vi "Main.vi"(11 "Module Admin":refnum<class "Delacor_lib_QMH_Cloneable Module Admin.lvclass">) -> ()   [LabVIEW 2020, in "Client HTTP Get.lvlib"]
doc: "This template is based off of the Queued Message Handler design pattern and the Queued Message Handler project template that ships with LabVIEW.\n\nThe main difference is that the queue is private to this module and communication between modules is performed via Broadcast and Request events.\n\nRequest events are wrapped in public API methods and are handled in the Event Handling Loop (EHL) of this VI. Any module can register for Broadcast events sent by this module. The EHL generates messages based on user interface actions.\n\nThe Message Handling Loop (MHL) processes messages generated by the EHL, or by other messages. The messages are string values, so new messages can be added easily to the Message Cases case structure in the MHL. Each message cluster can also provide an optional value for Message Data, which is a variant that can be converted to whatever message-specific data is required.\n_____\nBased on DQMH Project Template 6.0.0.91."
uses:
  Client HTTP Get.lvlib
  <vilib>/Delacor/Delacor QMH/Libraries/Cloneable Module Admin_class/Delacor_lib_QMH_Cloneable Module Admin.lvclass
  C:/Program Files (x86)/National Instruments/LabVIEW 2020/vi.lib/Delacor/Delacor QMH/Libraries/Module Admin_class/Delacor_lib_QMH_Module Admin.lvclass
  Module Data--cluster.ctl
  Do Something Argument--cluster.ctl
  <vilib>/Delacor/Delacor QMH/Libraries/Message Queue_class/Delacor_lib_QMH_Message Queue.lvclass/Delacor_lib_QMH_Message Queue.ctl
  Do Something Else Argument--cluster.ctl
  Do Something Else and Wait for Reply Argument--cluster.ctl
  Do Something Else and Wait (Reply Payload)--cluster.ctl
  <vilib>/Delacor/Delacor QMH/Libraries/Cloneable Module Admin_class/Delacor_lib_QMH_Cloneable Module Admin.lvclass/Delacor_lib_QMH_Cloneable Module Admin.ctl
  Stop Argument--cluster.ctl
  <vilib>/Delacor/Delacor QMH/Libraries/Module Admin_class/Delacor_lib_QMH_Module Admin.lvclass/Delacor_lib_QMH_Module Admin.ctl
  <vilib>/Delacor/Delacor QMH/Libraries/Message Queue_class/Delacor_lib_QMH_Enqueue Message (Single).vi
  <vilib>/Delacor/Delacor QMH/Libraries/Cloneable Module Admin_class/Delacor_lib_QMH_Get Module ID.vi
  <vilib>/Delacor/Delacor QMH/Libraries/Module Admin_class/Delacor_lib_QMH_Get External Launch.vi
  <vilib>/Utility/error.llb/Error Cluster From Error Code.vi
  <vilib>/ErrorRing/Error Ring.xnode
  <vilib>/Delacor/Delacor QMH/Libraries/Message Queue_class/Delacor_lib_QMH_Message Queue.lvclass
  <vilib>/httpClient/LabVIEWHTTPClient.lvlib
panel:
  out "Array Data GET *-HTTP":dbl[](array[numeric])
  out "body":string[](array[string])
  out "headers":string[](array[string])
  in  "#Variables":enum16{"1", "2", "3", "4", "5"}(ring)
  in  "Recibir":bool
  in  "GET":T1={"URL"="things.ubidots.com/api/v1.6/devices/system_daq/variable/values", "Nombre - Variable"="", "Token"="BBFF-FQubfN2B9slUP8xWYB99mULTCcM9aX"}
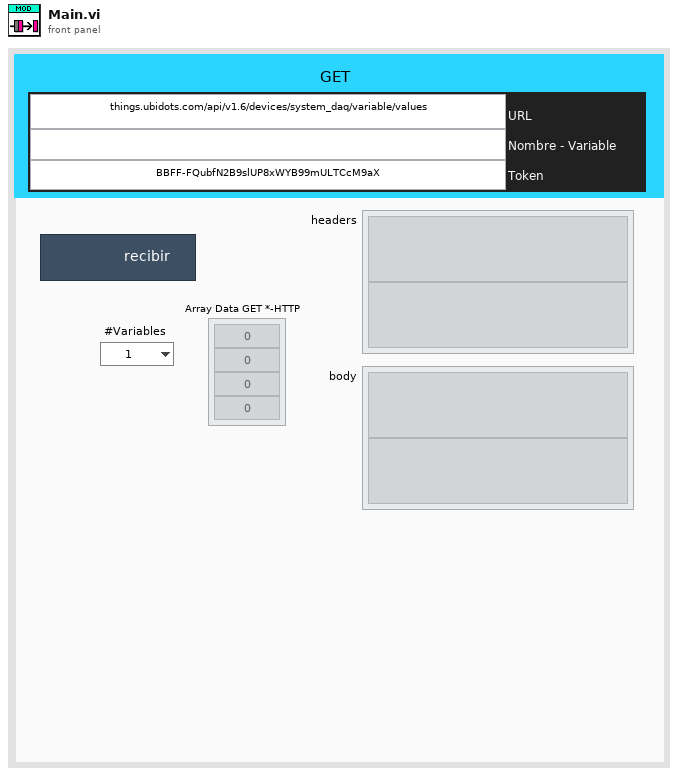
[diagram p1: front panel]
types:
  T1 = cluster{"URL":string, "Nombre - Variable":string, "Token":string}
  T2 = typedef "Client HTTP Get.lvlib/Request Events--cluster.ctl" = cluster{"Stop Module":refnum<user-event>, "Do Something":refnum<user-event>, "Do Something Else":refnum<user-event>, "Do Something Else and Wait for Reply":refnum<user-event>, "Show Panel":refnum<user-event>, "Hide Panel":refnum<user-event>, "Show Diagram":refnum<user-event>, "Get Module Execution Status":refnum<user-event>}
  T3 = typedef "Client HTTP Get.lvlib/Module Data--cluster.ctl" = cluster{"Status":string, "Body":string[]}
  T4 = typedef "Client HTTP Get.lvlib/Do Something Argument--cluster.ctl" = cluster{"Module ID":i32, "Do Something Msg":string}
  T5 = typedef "Client HTTP Get.lvlib/Do Something Else Argument--cluster.ctl" = cluster{"Module ID":i32, "Do Something Else Msg":string, "X":dbl}
  T6 = typedef "Client HTTP Get.lvlib/Do Something Else and Wait for Reply Argument--cluster.ctl" = cluster{"Module ID":i32, "Do Something Else Msg":string, "X":dbl, "Wait Notifier":refnum<notifier>, "wait for reply":bool}
  T7 = enum32{"invalid lock state", "Not Locked", "Locked (No Password)", "Password-protected"}
  T8 = typedef "Client HTTP Get.lvlib/Stop Argument--cluster.ctl" = cluster{"Module ID":i32, "Origin":string, "Exit via Stop Module Req?":bool, "Wait for Module to stop?":bool}
  T9 = enum32{"Invalid", "Standard", "Closed", "Hidden", "Minimized", "Maximized"}
  T10 = typedef "Client HTTP Get.lvlib/Do Something Else and Wait (Reply Payload)--cluster.ctl" = cluster{"Value":dbl, "error":errorcluster}
  T11 = typedef "LabVIEWHTTPClient.lvlib/ClientHandle.ctl" = refnum<k1>
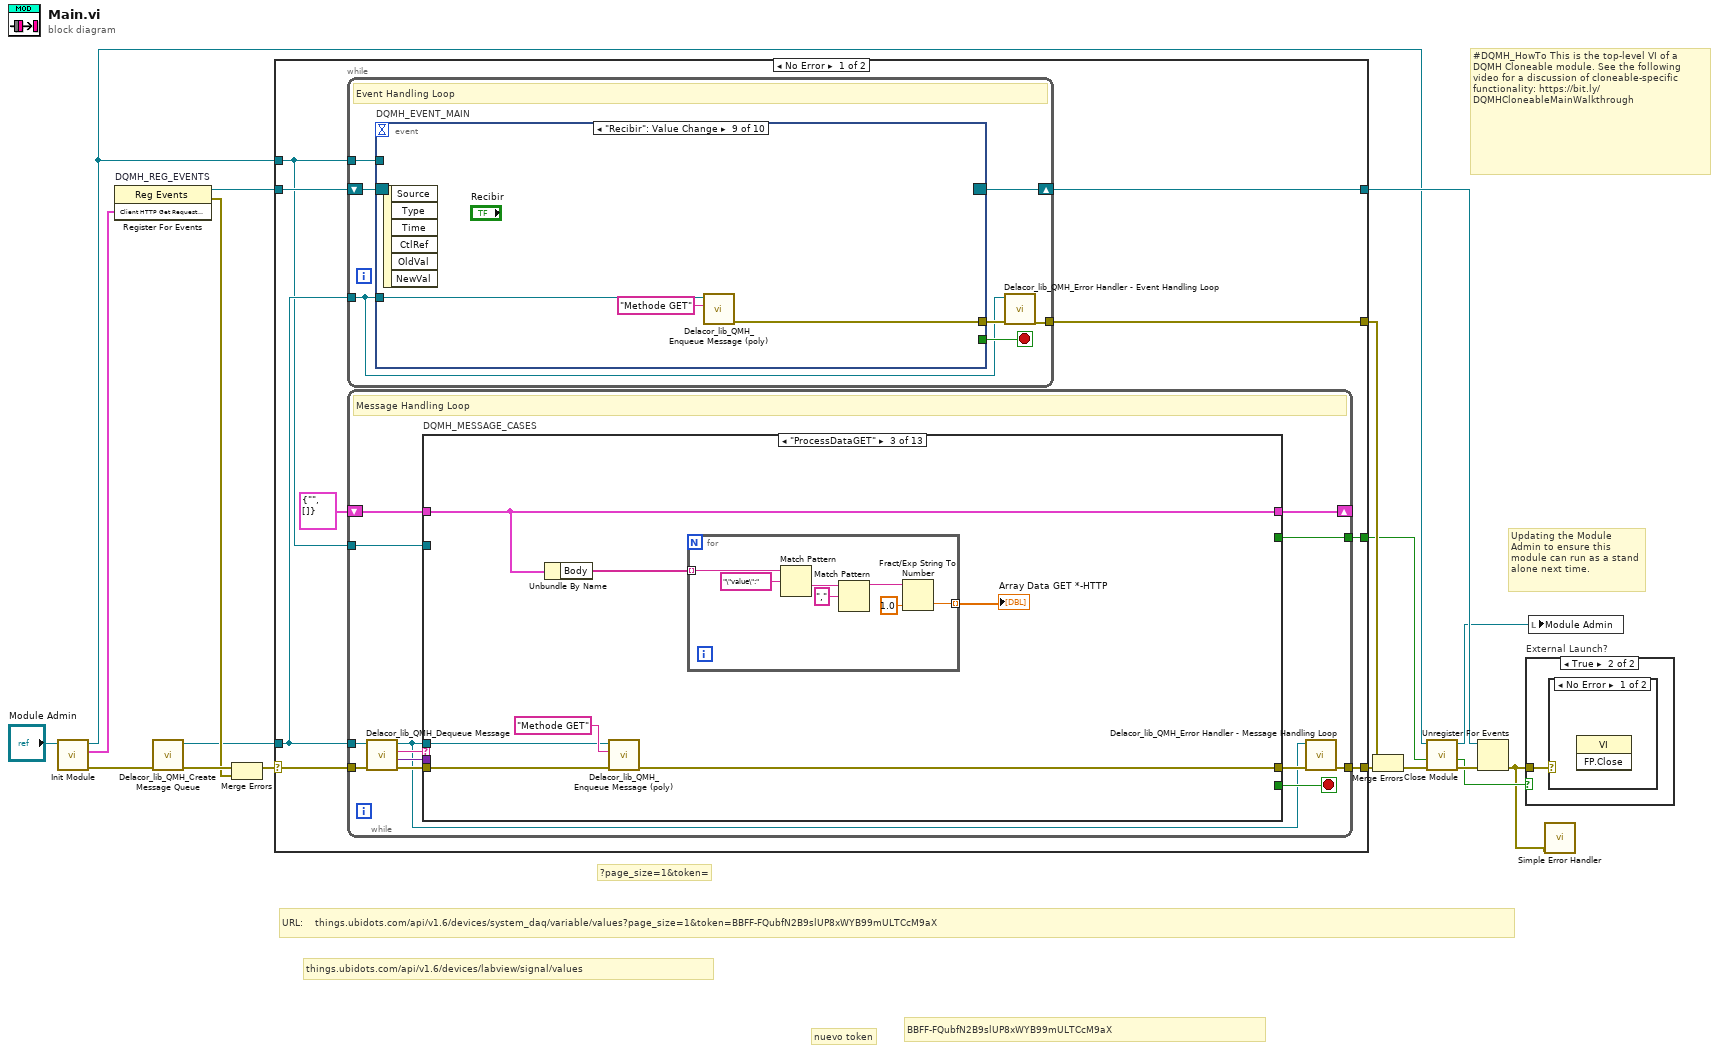
[diagram p0: block diagram]
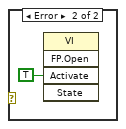
[diagram p3: hidden frame]
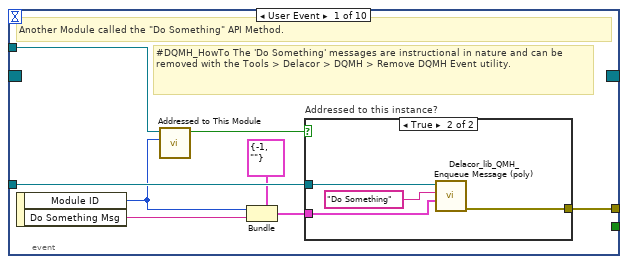
[diagram p4: hidden frame]
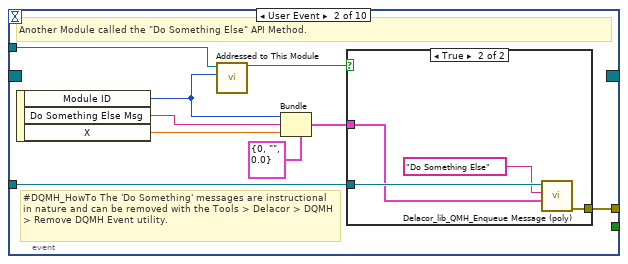
[diagram p6: hidden frame]
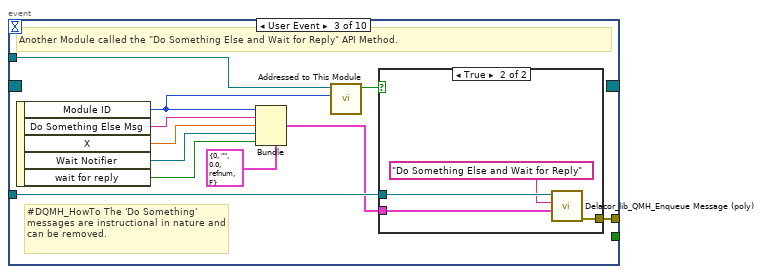
[diagram p8: hidden frame]
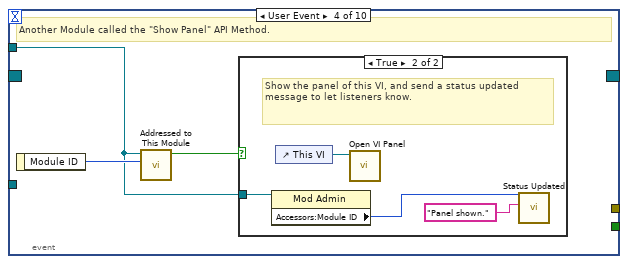
[diagram p10: hidden frame]
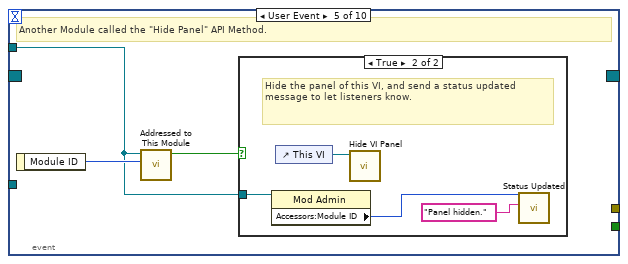
[diagram p12: hidden frame]
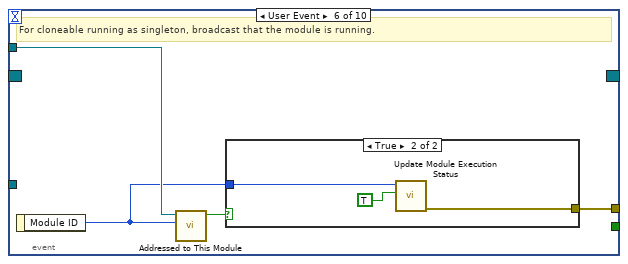
[diagram p14: hidden frame]
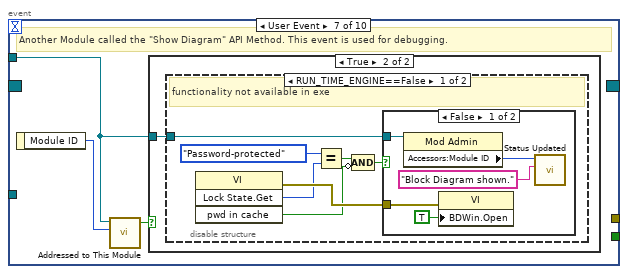
[diagram p16: hidden frame]
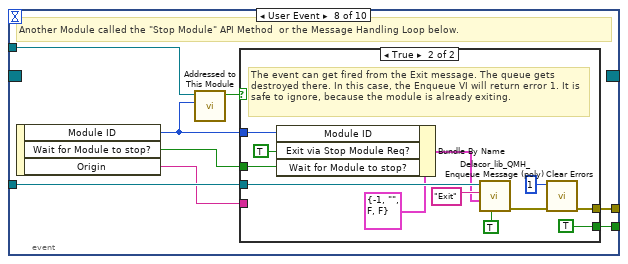
[diagram p20: hidden frame]
diagram:
  # "BBFF-FQubfN2B9slUP8xWYB99mULTCcM9aX"
  # "nuevo token"
  # "things.ubidots.com/api/v1.6/devices/labview/signal/values"
  # "URL:    things.ubidots.com/api/v1.6/devices/system_daq/variable/values?page_size=1&token=BBFF-FQubfN2B9slUP8xWYB99mULTCcM9aX"
  # "?page_size=1&token="
  # "#DQMH_HowTo This is the top-level VI of a DQMH Cloneable module. See the following video for a discussion of cloneable-specific functionality: https://bit.ly/DQMHCloneableMainWalkthrough"
  # "Updating the Module Admin to ensure this module can run as a stand alone next time."
  n1 = call "Init Module.vi"("Cloneable Module Admin in"="Module Admin") -> ("error out"=w15:errorcluster, "Client HTTP Get Request Events"=w8:T2, "Cloneable Module Admin out"=w5:refnum<class "Delacor_lib_QMH_Cloneable Module Admin.lvclass">)  [unwired: 8 in]
  n2 = register-events "DQMH_REG_EVENTS"(w8) -> (reference out=w9:refnum<event-registration>, error out=w11:errorcluster)  [unwired: 2 in]
  n3 = call <vilib>:"Delacor_lib_QMH_Create Message Queue.vi"("error in"=w15) -> ("error out"=w13:errorcluster, "Message Queue"=w7:refnum<class "Delacor_lib_QMH_Message Queue.lvclass">)  [unwired: 9 in]
  n4 = Merge Errors(w13, w11) -> (w12:errorcluster)
  n5 = case shown="No Error" w12 {
    selector: w12 -> [w25 w364]
    tunnel: [w27 w363] -> w16
    tunnel: [w24 w371] -> w10
    tunnel: w9 -> [w22 w371]
    tunnel: w7 -> [w21 w362]
    tunnel: [w26 _] -> w17
    tunnel: w5 -> [w20 w367]
    tunnel: [w19 _] -> w3
    frame No Error {
      n6 = while {
        tunnel: w21 -> [w28]
        shift-right: [w31] -> w24
        shift-left: w22 -> [w32]
        tunnel: [w33] -> w26
        tunnel: w20 -> [w29]
        stop <- w30 stop-if-true
        # "Event Handling Loop"
        n7 = event "DQMH_EVENT_MAIN" shown="[8] \"Recibir\": Value Change" {
          selector: w32 -> [_ _ _ _ _ _ _ _ _ _]
          dyn-events: [_ _ _ _ _ _ _ _ _ _] -> w31
          timeout: _ -> [_ _ _ _ _ _ _ _ _ _]
          tunnel: [_ _ _ _ _ _ _ w115 _ _] -> w30
          tunnel: w28 -> [w41 w54 w69 _ _ _ _ w118 w133 w136]
          tunnel: [w42 w55 w70 _ _ w92 _ w119 w134 w139] -> w34
          tunnel: w29 -> [w39 w52 w67 w75 w82 w90 w96 w117 _ w137]
          event User Event {
            # "#DQMH_HowTo The 'Do Something' messages are instructional in nature and can be removed with the Tools > Delacor > DQMH > Remove DQMH Event utility."
            # "Another Module called the \"Do Something\" API Method."
            n8 = event-data() -> ("Module ID"=w36:i32, "Do Something Msg"=w35:string)  [unwired: 1 in]
            n9 = call "Addressed to This Module.vi"("Module ID from Argument"=w36, "Module Admin"=w39) -> ("Addressed to this instance?"=w40:bool)  [unwired: 8 in, 1 out]
            n10 = Bundle(cluster=T4 {"Module ID"=-1, "Do Something Msg"=""} ("Do Something Argument"), "Module ID"=w36, "Do Something Msg"=w35) -> (w38:T4)
            n11 = case "Addressed to this instance?" shown="True" w40 {
              tunnel: w41 -> [_ w45]
              tunnel: [_ w46] -> w42
              tunnel: w38 -> [_ w43]
              frame False {
                # "Do nothing"
              }
              frame True {
                n12 = call-poly <vilib>:"Delacor_lib_QMH_Enqueue Message (poly).vi"("Message Data"=w43, "Message"="Do Something", "Message Queue in"=w45) -> ("error out"=w46:errorcluster)  [unwired: 7 in, 1 out]
              }
            }
          }
          event User Event {
            # "#DQMH_HowTo The 'Do Something' messages are instructional in nature and can be removed with the Tools > Delacor > DQMH > Remove DQMH Event utility."
            # "Another Module called the \"Do Something Else\" API Method."
            n13 = event-data() -> ("Module ID"=w47:i32, "Do Something Else Msg"=w48:string, "X"=w50:dbl)  [unwired: 1 in]
            n14 = call "Addressed to This Module.vi"("Module ID from Argument"=w47, "Module Admin"=w52) -> ("Addressed to this instance?"=w53:bool)  [unwired: 8 in, 1 out]
            n15 = Bundle(cluster=T5 {"Module ID"=0, "Do Something Else Msg"="", "X"=0.0} ("Do Something Else Argument"), "Module ID"=w47, "Do Something Else Msg"=w48, "X"=w50) -> (w49:T5)
            n16 = case shown="True" w53 {
              tunnel: w54 -> [_ w58]
              tunnel: [_ w59] -> w55
              tunnel: w49 -> [_ w56]
              frame False {
              }
              frame True {
                n17 = call-poly <vilib>:"Delacor_lib_QMH_Enqueue Message (poly).vi"("Message Data"=w56, "Message"="Do Something Else", "Message Queue in"=w58) -> ("error out"=w59:errorcluster)  [unwired: 7 in, 1 out]
              }
            }
          }
          event User Event {
            # "#DQMH_HowTo The 'Do Something' messages are instructional in nature and can be removed."
            # "Another Module called the \"Do Something Else and Wait for Reply\" API Method."
            n18 = event-data() -> ("Module ID"=w65:i32, "Do Something Else Msg"=w63:string, "X"=w62:dbl, "Wait Notifier"=w61:refnum<notifier>, "wait for reply"=w60:bool)  [unwired: 1 in]
            n19 = Bundle(cluster=T6 {"Module ID"=0, "Do Something Else Msg"="", "X"=0.0, "Wait Notifier"=refnum, "wait for reply"=FALSE} ("Do Something Else and Wait for Reply Argument"), "Module ID"=w65, "Do Something Else Msg"=w63, "X"=w62, "Wait Notifier"=w61, "wait for reply"=w60) -> (w64:T6)
            n20 = call "Addressed to This Module.vi"("Module ID from Argument"=w65, "Module Admin"=w67) -> ("Addressed to this instance?"=w68:bool)  [unwired: 8 in, 1 out]
            n21 = case shown="True" w68 {
              tunnel: [_ w74] -> w70
              tunnel: w69 -> [_ w73]
              tunnel: w64 -> [_ w71]
              frame False {
              }
              frame True {
                n22 = call-poly <vilib>:"Delacor_lib_QMH_Enqueue Message (poly).vi"("Message Data"=w71, "Message"="Do Something Else and Wait for Reply", "Message Queue in"=w73) -> ("error out"=w74:errorcluster)  [unwired: 7 in, 1 out]
              }
            }
          }
          event User Event {
            # "Another Module called the \"Show Panel\" API Method."
            n23 = event-data() -> ("Module ID"=w76:i32)  [unwired: 1 in]
            n24 = call "Addressed to This Module.vi"("Module ID from Argument"=w76, "Module Admin"=w75) -> ("Addressed to this instance?"=w77:bool)  [unwired: 8 in, 1 out]
            n25 = case shown="True" w77 {
              tunnel: w75 -> [_ w79]
              frame False {
              }
              frame True {
                # "Show the panel of this VI, and send a status updated message to let listeners know."
                n26 = property class="Mod Admin"(reference=w79) -> ("Accessors:Module ID"=w78:i32)  [unwired: 1 in, 2 out]
                n27 = control-ref of="This VI"() -> (w81:refnum<vi>)
                n28 = call "Open VI Panel.vi"("VI"=w81) -> ()  [unwired: 10 in, 1 out]
                n29 = call "Status Updated.vi"("Status"="Panel shown." ("format string"), "Module ID"=w78) -> ()  [unwired: 9 in, 1 out]
              }
            }
          }
          event User Event {
            # "Another Module called the \"Hide Panel\" API Method."
            n30 = event-data() -> ("Module ID"=w83:i32)  [unwired: 1 in]
            n31 = call "Addressed to This Module.vi"("Module ID from Argument"=w83, "Module Admin"=w82) -> ("Addressed to this instance?"=w84:bool)  [unwired: 8 in, 1 out]
            n32 = case shown="True" w84 {
              tunnel: w82 -> [_ w86]
              frame False {
              }
              frame True {
                # "Hide the panel of this VI, and send a status updated message to let listeners know."
                n33 = property class="Mod Admin"(reference=w86) -> ("Accessors:Module ID"=w85:i32)  [unwired: 1 in, 2 out]
                n34 = control-ref of="This VI"() -> (w88:refnum<vi>)
                n35 = call "Hide VI Panel.vi"("VI"=w88) -> ()  [unwired: 10 in, 1 out]
                n36 = call "Status Updated.vi"("Status"="Panel hidden." ("format string"), "Module ID"=w85) -> ()  [unwired: 9 in, 1 out]
              }
            }
          }
          event User Event {
            # "For cloneable running as singleton, broadcast that the module is running."
            n37 = event-data() -> ("Module ID"=w89:i32)  [unwired: 1 in]
            n38 = call "Addressed to This Module.vi"("Module ID from Argument"=w89, "Module Admin"=w90) -> ("Addressed to this instance?"=w91:bool)  [unwired: 8 in, 1 out]
            n39 = case shown="True" w91 {
              tunnel: [_ w95] -> w92
              tunnel: w89 -> [_ w94]
              frame False {
              }
              frame True {
                n40 = call "Update Module Execution Status.vi"("Running?"=TRUE, "Module ID"=w94) -> ("error out"=w95:errorcluster)  [unwired: 9 in]
              }
            }
          }
          event User Event {
            # "Another Module called the \"Show Diagram\" API Method. This event is used for debugging."
            n41 = event-data() -> ("Module ID"=w97:i32)  [unwired: 1 in]
            n42 = call "Addressed to This Module.vi"("Module ID from Argument"=w97, "Module Admin"=w96) -> ("Addressed to this instance?"=w98:bool)  [unwired: 8 in, 1 out]
            n43 = case shown="True" w98 {
              tunnel: w96 -> [_ w99]
              frame False {
              }
              frame True {
                n44 = disable-structure shown="RUN_TIME_ENGINE==False" {
                  disable-tunnel: w99 -> [w100 _]
                  frame condition #0 (active) {
                    # "functionality not available in exe"
                    n45 = invoke class="VI" method="Lock State.Get"() -> (error out=w106:errorcluster, "Get Lock State"=w105:T7, "pwd in cache"=w102:bool)  [unwired: 4 in, 1 out]
                    n46 = Equal?(x=T7."Password-protected", y=w105) -> (x = y?=w103:bool)
                    n47 = Compound Arithmetic op=AND(w103, invert w102) -> (w101:bool)
                    n48 = case shown="False" w101 {
                      tunnel: w106 -> [w111 _]
                      tunnel: w100 -> [w108 _]
                      frame False {
                        n49 = property class="Mod Admin"(reference=w108) -> ("Accessors:Module ID"=w107:i32)  [unwired: 1 in, 2 out]
                        n50 = property class="VI"(error in=w111, "BDWin.Open"=TRUE ("Block Diagram Window:Open")) -> ()  [unwired: 1 in, 2 out]
                        n51 = call "Status Updated.vi"("Status"="Block Diagram shown." ("format string"), "Module ID"=w107) -> ()  [unwired: 9 in, 1 out]
                      }
                      frame True {
                        # "Password-protected VI, and the password is not in the cache. Do not show the diagram."
                      }
                    }
                  }
                  frame condition #1 {
                  }
                }
              }
            }
          }
          event User Event {
            # "Another Module called the \"Stop Module\" API Method  or the Message Handling Loop below."
            n52 = event-data() -> ("Module ID"=w113:i32, "Wait for Module to stop?"=w114:bool, "Origin"=w112:string)  [unwired: 1 in]
            n53 = call "Addressed to This Module.vi"("Module ID from Argument"=w113, "Module Admin"=w117) -> ("Addressed to this instance?"=w116:bool)  [unwired: 8 in, 1 out]
            n54 = case shown="True" w116 {
              tunnel: [_ w130] -> w119
              tunnel: w118 -> [_ w126]
              tunnel: [_ TRUE] -> w115
              tunnel: w114 -> [_ w121]
              tunnel: w113 -> [_ w123]
              tunnel: w112 -> [_ _]
              frame False {
              }
              frame True {
                # "The event can get fired from the Exit message. The queue gets destroyed there. In this case, the Enqueue VI will return error 1. It is safe to ignore, because the module is already exiting."
                n55 = Bundle By Name(cluster=T8 {"Module ID"=-1, "Origin"="", "Exit via Stop Module Req?"=FALSE, "Wait for Module to stop?"=FALSE} ("Stop Argument"), "Module ID"=w123, "Exit via Stop Module Req?"=TRUE, "Wait for Module to stop?"=w121) -> (w120:T8)
                n56 = call-poly <vilib>:"Delacor_lib_QMH_Enqueue Message (poly).vi"("Priority Message? (F)"=TRUE, "Message Data"=w120, "Message"="Exit", "Message Queue in"=w126) -> ("error out"=w131:errorcluster)  [unwired: 6 in, 1 out]
                n57 = call <vilib>:"Clear Errors.vi"("error in (no error)"=w131, "specific error code to clear (0: all)"=1) -> ("error out"=w130:errorcluster)  [unwired: 4 in, 1 out]
              }
            }
          }
          event "Recibir": Value Change {
            n58 = event-data() -> ()  [unwired: 1 in, 6 out]
            n59 = call-poly <vilib>:"Delacor_lib_QMH_Enqueue Message (poly).vi"("Message"="Methode GET", "Message Queue in"=w133) -> ("error out"=w134:errorcluster)  [unwired: 8 in, 1 out]
          }
          event Panel Close? {
            w138 = TRUE  # Discard the event, the MHL is responsible for closing and stopping this VI.
            # "Hide the panel or send the 'Exit' message if the user clicks the 'X' on the module main VI panel."
            n60 = event-data() -> ()  [unwired: 1 in, 1 out]
            n61 = property class="Mod Admin"(reference=w137) -> ("Accessors:External Launch"=w135:bool)  [unwired: 1 in, 2 out]
            n62 = case shown="True" w135 {
              tunnel: w136 -> [_ w143]
              tunnel: [_ w144] -> w139
              frame True {
                # "If externally launched, clicking the 'X' hides the panel, but doesn't close it."
                n63 = control-ref of="This VI"() -> (w140:refnum<vi>)
                n64 = call "Hide VI Panel.vi"("VI"=w140) -> ()  [unwired: 10 in, 1 out]
              }
              frame False {
                # "If run as a stand-alone VI, clicking the panel 'X' stops the VI."
                n65 = call-poly <vilib>:"Delacor_lib_QMH_Enqueue Message (poly).vi"("Priority Message? (F)"=TRUE, "Message"="Exit", "Message Queue in"=w143) -> ("error out"=w144:errorcluster)  [unwired: 7 in, 1 out]
              }
            }
            n66 = event-data("Discard?"=w138) -> ()  [unwired: 1 in, 1 out]
          }
        }
        n67 = call-dynamic "Delacor_lib_QMH_Error Handler - Event Handling Loop.vi"("error in"=w34, "Message Queue in"=w28) -> ("dup error in"=w33:errorcluster)  [unwired: 8 in, 1 out]
      }
      n68 = while {
        tunnel: w21 -> [w148]
        shift-right: [w152] -> _
        shift-left: T3 {"Status"="", "Body"=[]} ("Data Cluster") -> [w153]
        tunnel: w25 -> [w156]
        tunnel: [w154] -> w27
        tunnel: w20 -> [w146]
        tunnel: [w145] -> w19
        stop <- w151 stop-if-true
        # "Message Handling Loop"
        n69 = call-dynamic "Delacor_lib_QMH_Dequeue Message.vi"("error in"=w156, "Message Queue in"=w148) -> ("error out"=w155:errorcluster, "Message Data"=w149:variant, "Message"=w150:string, "Message Queue out"=w147:refnum<class "Delacor_lib_QMH_Message Queue.lvclass">)  [unwired: 6 in]
        n70 = case "DQMH_MESSAGE_CASES" shown="\"ProcessDataGET\"" w150 {
          selector: w150 -> [_ _ _ _ _ _ _ _ _ _ _ _ w349]
          tunnel: w147 -> [_ w181 w227 _ _ _ _ _ _ w301 _ w339 _]
          tunnel: w155 -> [w172 w182 w229 w239 w249 w260 w281 w296 w298 w309 w322 w345 w351]
          tunnel: [w170 w180 w225 w239 w247 w259 w280 w295 w298 w299 w321 w342 w352] -> w157
          tunnel: w153 -> [w158 w179 w226 w238 w246 w258 w278 w294 w297 w305 w319 w338 w350]
          tunnel: [w158 w178 w226 w238 w246 w258 w278 w294 w297 w305 w319 w338 w350] -> w152
          tunnel: [_ _ _ _ _ _ _ _ _ _ _ w337 _] -> w151
          tunnel: w149 -> [_ _ _ _ w245 w255 w275 _ _ w304 _ w335 _]
          tunnel: w146 -> [w160 _ _ _ w241 w251 w265 _ _ w303 w317 w331 w347]
          tunnel: [_ _ _ _ _ _ _ _ _ _ _ w333 _] -> w145
          frame "Initialize" {
            # "Initialize - Any operation that needs to be done before the module can receive messages. Synchronize Caller Events.vi will inform Start Module.vi that the module has launched and is ready to receive messages. Module Did Init.vi will broadcast that the module initialized."
            n71 = call "Synchronize Caller Events.vi"("error in (no error)"=w172, "Module Admin"=w160) -> ("error out"=w171:errorcluster, "Module Admin out"=w159:refnum<class "Delacor_lib_QMH_Cloneable Module Admin.lvclass">)  [unwired: 8 in]
            n72 = property class="Mod Admin"(reference=w159) -> ("Accessors:Module ID"=w162:i32, "Accessors:External Launch"=w161:bool)  [unwired: 1 in, 2 out]
            n73 = call "Module Name--constant.vi"("Module ID"=w162) -> ("Module Name"=w168:string)  [unwired: 10 in]
            n74 = property class="VI"("Front Panel.Title"=w168) -> (reference out=w169:refnum<vi>, error out=w173:errorcluster)  [unwired: 2 in]
            n75 = Select(t=T9."Hidden" ("State"), s=w161, f=T9."Standard" ("State")) -> (s? t:f=w165:T9)
            n76 = invoke class="VI" method="FP.Open"(reference=w169, error in=w173, "State"=w165) -> ()  [unwired: 2 in, 5 out]
            n77 = call "Module Name--constant.vi"("Module ID"=w162) -> ("Module Name"=w163:string)  [unwired: 10 in]
            n78 = call "Module Did Init.vi"("error in (no error)"=w171, "Initialized?"=TRUE, "Origin"=w163, "Module ID"=w162) -> ("error out"=w170:errorcluster)  [unwired: 7 in]
          }
          frame "Methode GET" {
            n79 = Unbundle By Name("GET") -> ("URL"=w201:string, "Token"=w197:string)  [unwired: 1 out]
            n80 = call <vilib>:"OpenHandle.vi"("error in (no error)"=w182) -> ("client handle out"=w189:T11, "error out"=w190:errorcluster)  [unwired: 13 in]
            n81 = call <vilib>:"AddHeader.vi"("client handle"=w189, "header"="Content-Type", "value"="application/json", "error in (no error)"=w190) -> ("client handle out"=w191:T11, "error out"=w192:errorcluster)  [unwired: 10 in]
            n82 = Concatenate Strings("?page_size=1&token=" ("string"), w197) -> (w200:string)
            n83 = Match Pattern(string=w201, regular expression="/system_daq/") -> (before substring=w203:string, match substring=w202:string, after substring=w195:string)  [unwired: 1 in, 1 out]
            n84 = case shown="\"1\", Default" "#Variables" {
              tunnel: [1 2 3 4 5] -> w199
              frame "1", Default {
              }
              frame "2" {
              }
              frame "3" {
              }
              frame "4" {
              }
              frame "5" {
              }
            }
            n85 = Match Pattern(string=w195, regular expression="/values") -> (before substring=w196:string)  [unwired: 1 in, 3 out]
            n86 = for {
              N: w199 -> [_]
              tunnel: w192 -> [w222]
              tunnel: [w221] -> w193
              tunnel: w191 -> [w223]
              tunnel: [w220] -> w194
              tunnel: w196 -> [w218]
              tunnel: [w215] -> w174 mode=indexing
              tunnel: [w214] -> w175 mode=indexing
              tunnel: w203 -> [w212]
              tunnel: w200 -> [w209]
              tunnel: w202 -> [w211]
              i -> [w219]
              n87 = Increment(x=w219) -> (x+1=w217:i32)
              n88 = Number To Decimal String(number=w217) -> (decimal integer string=w216:string)  [unwired: 1 in]
              n89 = Concatenate Strings(w218, w216) -> (w210:string)
              n90 = Concatenate Strings(w212, w211, w210, w209) -> (w213:string)
              n91 = call <vilib>:"GET.vi"("client handle"=w223, "url"=w213, "error in (no error)"=w222) -> ("client handle out"=w220:T11, "headers"=w215:string, "body"=w214:string, "error out"=w221:errorcluster)  [unwired: 9 in]
            }
            "body" <- w175
            "headers" <- w174
            n92 = call <vilib>:"CloseHandle.vi"("client handle"=w194, "error in (no error)"=w193) -> ("error out"=w198:errorcluster)  [unwired: 13 in]
            n93 = Bundle By Name(cluster=w179, "Body"=w175) -> (w178:T3)
            n94 = call-poly <vilib>:"Delacor_lib_QMH_Enqueue Message (poly).vi"("error in"=w198, "Message"="ProcessDataGET", "Message Queue in"=w181) -> ("error out"=w180:errorcluster)  [unwired: 7 in, 1 out]
          }
          frame "ProcessDataGET" {
            n95 = Unbundle By Name(w226) -> ("Body"=w230:string[])
            n96 = call-poly <vilib>:"Delacor_lib_QMH_Enqueue Message (poly).vi"("error in"=w229, "Message"="Methode GET", "Message Queue in"=w227) -> ("error out"=w225:errorcluster)  [unwired: 7 in, 1 out]
            n97 = for {
              tunnel: w230 -> [w237] mode=indexing
              tunnel: [w231] -> w224 mode=indexing
              n98 = Match Pattern(string=w237, regular expression="\"value\":") -> (after substring=w235:string)  [unwired: 1 in, 3 out]
              n99 = Match Pattern(string=w235, regular expression=",") -> (before substring=w233:string)  [unwired: 1 in, 3 out]
              n100 = Fract/Exp String To Number(string=w233, default (0 dbl)=1.0 ("default (0 DBL)")) -> (number=w231:dbl)  [unwired: 2 in, 1 out]
            }
            "Array Data GET *-HTTP" <- w224
          }
          frame "---Module Specific---" {
            # "Separator -- The following cases handle messages specific to this Module."
          }
          frame "Do Something" {
            # "#DQMH_HowTo The 'Do Something' messages are instructional in nature and can be removed with the Tools > Delacor > DQMH > Remove DQMH Event utility."
            # "Do Something - Replace this message with functionality for your own application. Note that this message also fires the \"Did Something\" broadcast event."
            n101 = Variant To Data(error in=w249, type=T4 {"Module ID"=-1, "Do Something Msg"=""} ("Do Something Argument"), Variant=w245) -> (data=w244:T4, error out=w248:errorcluster)
            n102 = property class="Mod Admin"(reference=w241) -> ("Accessors:Module ID"=w240:i32)  [unwired: 1 in, 2 out]
            n103 = Unbundle By Name(w244) -> ("Do Something Msg"=w242:string)
            n104 = call "Status Updated.vi"("Status"=w242, "Module ID"=w240) -> ()  [unwired: 9 in, 1 out]
            n105 = call "Did Something.vi"("error in (no error)"=w248, "Did Something Msg"=w242, "Module ID"=w240) -> ("error out"=w247:errorcluster)  [unwired: 8 in]
          }
          frame "Do Something Else" {
            # "#DQMH_HowTo The 'Do Something' messages are instructional in nature and can be removed with the Tools > Delacor > DQMH > Remove DQMH Event utility."
            # "Do Something Else - Replace this message with functionality for your own application."
            n106 = Variant To Data(error in=w260, type=T5 {"Module ID"=0, "Do Something Else Msg"="", "X"=0.0} ("Do Something Else Argument"), Variant=w255) -> (data=w256:T5, error out=w259:errorcluster)
            n107 = Unbundle By Name(w256) -> ("Do Something Else Msg"=w254:string, "X"=w253:dbl)
            n108 = property class="Mod Admin"(reference=w251) -> ("Accessors:Module ID"=w250:i32)  [unwired: 1 in, 2 out]
            n109 = Format Into String(initial string=w254, w253) -> (resulting string=w252:string)  [unwired: 2 in, 1 out]
            n110 = call "Status Updated.vi"("Status"=w252, "Module ID"=w250) -> ()  [unwired: 9 in, 1 out]
          }
          frame "Do Something Else and Wait for Reply" {
            w268 = "X(%.2f)+Offset(%.2f)=%.2f"  # status message format string
            # "#DQMH_HowTo The 'Do Something' messages are instructional in nature and can be removed."
            # "Send back X with a random offset"
            # "Do Something Else and Wait for Reply - Replace this message with functionality for your own application. Note that this message must fire a notifier to let callers know it has finished execution, and it returns an error if the 'Value' is negative."
            n111 = Variant To Data(error in=w281, type=T6 {"Module ID"=0, "Do Something Else Msg"="", "X"=0.0, "Wait Notifier"=refnum, "wait for reply"=FALSE} ("Do Something Else and Wait for Reply Argument"), Variant=w275) -> (data=w276:T6, error out=w262:errorcluster)
            n112 = Unbundle By Name(w276) -> ("Wait Notifier"=w273:refnum<notifier>, "Do Something Else Msg"=w274:string, "X"=w270:dbl, "wait for reply"=w261:bool)
            n113 = property class="Mod Admin"(reference=w265) -> ("Accessors:Module ID"=w264:i32)  [unwired: 1 in, 2 out]
            n114 = Random Number (0-1)() -> (number: 0 to 1=w269:dbl)
            n115 = Add(x=w269, y=w270) -> (x+y=w263:dbl)
            n116 = Format Into String(format string=w268, initial string=w274, w270, w269, w263) -> (resulting string=w266:string)  [unwired: 1 in, 1 out]
            n117 = Less Than 0?(x=w263) -> (x < 0?=w267:bool)
            n118 = case shown="True" w267 {
              tunnel: [_ w288] -> w279
              frame False {
              }
              frame True {
                n119 = xnode "Error Ring"() -> ("error out"=w288:errorcluster)
              }
            }
            n120 = Bundle By Name(cluster=T10 {"Value"=0.0, "error"={"status"=FALSE, "code"=0, "source"=""}} ("notification"), "error"=w279, "Value"=w263) -> (w271:T10)
            n121 = call "Status Updated.vi"("Status"=w266, "Module ID"=w264) -> ()  [unwired: 9 in, 1 out]
            n122 = case shown="True" w261 {
              tunnel: w273 -> [_ w285]
              tunnel: w271 -> [_ w284]
              frame False {
              }
              frame True {
                # "Simulate an operation that requires a wait."
                n123 = Wait (ms)(milliseconds to wait=u32 1000) -> (millisecond timer value=w282:u32)
                n124 = flat-sequence {
                  tunnel: w285 -> [w287]
                  tunnel: w284 -> [w286]
                  tunnel: w282 -> [_]
                  frame #0 {
                    n125 = Send Notification(notification=w286, notifier=w287) -> ()  [unwired: 1 in, 2 out]
                  }
                }
              }
            }
            n126 = Merge Errors(w262, w279) -> (w280:errorcluster)
          }
          frame "---Copy This Frame---" {
            # "Duplicate this frame when creating new messages.  Change this comment in the duplicated frame to describe this message."
            n127 = Merge Errors(w296) -> (w295:errorcluster)
          }
          frame "---Exit and Error Handling---" {
            # "Separator - the following cases handle errors and exit messages."
          }
          frame "Error" {
            # "Error - Check the error message data and respond accordingly. This message is sent by the \"Error Handler\" VIs at the end of each loop in this application."
            n128 = property class="Mod Admin"(reference=w303) -> ("Accessors:External Launch"=w302:bool, "Accessors:Module ID"=w300:i32)  [unwired: 1 in, 2 out]
            n129 = Variant To Data(error in=w309, type=errorcluster {"status"=FALSE, "code"=0, "source"=""} ("error constant"), Variant=w304) -> (data=w310:errorcluster, error out=w307:errorcluster)
            n130 = call "Error Reported.vi"("Error"=w310, "Module ID"=w300) -> ()  [unwired: 9 in, 1 out]
            n131 = case shown="False" w302 {
              tunnel: [w315 _] -> w306
              tunnel: w301 -> [w313 _]
              tunnel: w310 -> [w314 _]
              frame False {
                # "If the module is running standalone, then pop up an error dialog and call the \"Exit\" message."
                n132 = call <vilib>:"Simple Error Handler.vi"("error in (no error)"=w314) -> ()  [unwired: 4 in, 5 out]
                n133 = call-poly <vilib>:"Delacor_lib_QMH_Enqueue Message (poly).vi"("Priority Message? (F)"=TRUE, "Message"="Exit", "Message Queue in"=w313) -> ("error out"=w315:errorcluster)  [unwired: 7 in, 1 out]
              }
              frame True {
                # "If the module was launched externally, calling the Error Reported broadcast VI is the only action performed by the \"Error\" message. The module's caller can then process the error appropriately."
              }
            }
            n134 = Merge Errors(w307, w306) -> (w299:errorcluster)
            n135 = call <vilib>:"Simple Error Handler.vi"("error in (no error)"=w299) -> ()  [unwired: 4 in, 5 out]
          }
          frame "Simulate MHL Error" {
            # "#DQMH_HowTo The 'Simulate MHL Error' button  illustrates how the MHL handles errors. This event is instructional in nature and can be removed."
            # "Simulate an error occurring at the MHL"
            n136 = property class="Mod Admin"(reference=w317) -> ("Accessors:Module ID"=w318:i32)  [unwired: 1 in, 2 out]
            n137 = call "Module Name--constant.vi"("Module ID"=w318) -> ("Module Name"=w316:string)  [unwired: 10 in]
            n138 = xnode "Error Ring"("parameter 0"=w316) -> ("error out"=w320:errorcluster)
            n139 = Merge Errors(w322, w320) -> (w321:errorcluster)
          }
          frame "Exit" {
            w336 = 91  # 91: not all Exit messages will have an argument
            w337 = TRUE  # Stop the VI
            # "Release the message queue reference"
            # "#CodeNeeded - Add any required cleanup code here."
            # "Exit - Exit the application."
            n140 = Variant To Data(error in=w345, type=T8 {"Module ID"=-1, "Origin"="", "Exit via Stop Module Req?"=FALSE, "Wait for Module to stop?"=FALSE} ("Stop Argument"), Variant=w335) -> (data=w332:T8, error out=w340:errorcluster)
            n141 = call <vilib>:"Clear Errors.vi"("error in (no error)"=w340, "specific error code to clear (0: all)"=w336) -> ("error out"=w344:errorcluster)  [unwired: 4 in, 1 out]
            n142 = control-ref of="This VI"() -> (w330:refnum<vi>)
            n143 = call-dynamic "Delacor_lib_QMH_Release Message Queue.vi"("error in"=w344, "Message Queue"=w339) -> ("error out"=w343:errorcluster)  [unwired: 9 in]
            n144 = call "Handle Exit.vi"("Stop Argument"=w332, "Module Admin in"=w331, "VI reference"=w330) -> ("error out"=w341:errorcluster, "Wait for Stop?"=w333:bool)  [unwired: 7 in]
            n145 = Merge Errors(w343, w341) -> (w342:errorcluster)
          }
          frame Default {
            # "'Default' case only runs if there is a message that isn't defined in any of the other cases.  Output a programming error."
            n146 = property class="Mod Admin"(reference=w347) -> ("Accessors:Module ID"=w346:i32)  [unwired: 1 in, 2 out]
            n147 = call "Module Name--constant.vi"("Module ID"=w346) -> ("Module Name"=w348:string)  [unwired: 10 in]
            n148 = xnode "Error Ring"("parameter 0"=w349, "parameter 1"=w348) -> ("error out"=w353:errorcluster)
            n149 = Merge Errors(w351, w353) -> (w352:errorcluster)
          }
        }
        n150 = call-dynamic "Delacor_lib_QMH_Error Handler - Message Handling Loop.vi"("error in"=w157, "Message Queue in"=w147) -> ("dup error in"=w154:errorcluster)  [unwired: 8 in, 1 out]
      }
    }
    frame Error {
      n151 = call "Synchronize Caller Events.vi"("Module Admin"=w367) -> ("Module Admin out"=w366:refnum<class "Delacor_lib_QMH_Cloneable Module Admin.lvclass">)  [unwired: 9 in, 1 out]
      n152 = property class="Mod Admin"(reference=w366) -> ("Accessors:Module ID"=w365:i32)  [unwired: 1 in, 2 out]
      n153 = call-dynamic "Delacor_lib_QMH_Release Message Queue.vi"("error in"=w364, "Message Queue"=w362) -> ("error out"=w363:errorcluster)  [unwired: 9 in]
      n154 = call "Module Name--constant.vi"("Module ID"=w365) -> ("Module Name"=w370:string)  [unwired: 10 in]
      n155 = Format Into String(format string="An error occurred during initialization. %s is no longer running.", w370) -> (resulting string=w368:string)  [unwired: 2 in, 1 out]
      n156 = call "Error Reported.vi"("Additional Information"=w368, "Error"=w363, "Module ID"=w365) -> ()  [unwired: 8 in, 1 out]
    }
  }
  n157 = Merge Errors(w17, w16) -> (w18:errorcluster)
  n158 = call "Close Module.vi"("error in"=w18, "Wait for stop?"=w3, "Module Admin in"=w5) -> ("error out"=w14:errorcluster, "External Launch"=w2:bool, "Module Admin out"=w4:refnum<class "Delacor_lib_QMH_Cloneable Module Admin.lvclass">)  [unwired: 6 in]
  n159 = Unregister For Events(event registration refnum=w10, error in=w14) -> (error out=w1:errorcluster)
  n160 = case "External Launch?" shown="True" w2 {
    tunnel: w1 -> [_ w372]
    frame False {
    }
    frame True {
      n161 = case shown="No Error" w372 {
        frame No Error {
          n162 = invoke class="VI" method="FP.Close"() -> ()  [unwired: 3 in, 3 out]
        }
        frame Error {
          n163 = invoke class="VI" method="FP.Open"("Activate"=TRUE ("Activate?")) -> ()  [unwired: 4 in, 5 out]
        }
      }
    }
  }
  n164 = local write "Module Admin"(w4) -> ()
  n165 = call <vilib>:"Simple Error Handler.vi"("error in (no error)"=w1) -> ()  [unwired: 4 in, 5 out]
